vi "Main Development.vi"() -> ()   [LabVIEW 2021]
doc: "This template is for the Queued Message Handler design pattern.\n\nThe Event Handling Loop generates messages based on user interface actions.\n\nThe Message Handling Loop processes messages generated by the Event Handling Loop, or by other messages. The messages are string values, so new messages can be added easily to the Message Cases case structure in the Message Handling Loop. Each message cluster can also provide an optional value for Message Data, which is a variant that can be converted to whatever message-specific data is required."
uses:
  controls/UI Data.ctl
  support/Message Queue/Enqueue Message (Single).vi
  <vilib>/Utility/error.llb/Error Cluster From Error Code.vi
  <vilib>/ErrorRing/Error Ring.xnode
  support/Message Queue/Message Queue.lvlib
  support/User Event - Stop/User Event - Stop.lvlib
panel:
  out "Logging Clock":bool
  out "Sampling Clock":bool
  out "Logging Active":bool
  out "Log Delay":u32
  in  "Log Frequency (Hz)":dbl=2.0 min=0.0 step=1.0
  out "Sampling State":string(combo)="Paused"
  out "Pressure (bar)":dbl
  out "Pressure Chart":dbl(graph)
  out "Runtime Error out":errorcluster
  out "Measured Voltage":dbl format="%0.2f"
  out "Sample Delay mS":u32
  out "Logging State":string(combo)="Paused"
  out "Sampling Active":bool
  in  "Sample Rate (Hz)":dbl=10.0 min=0.0 step=1.0
  out "Program State":string
  in  "Start Logging":bool
  in  "Start Sampling":bool
  in  "Exit":bool
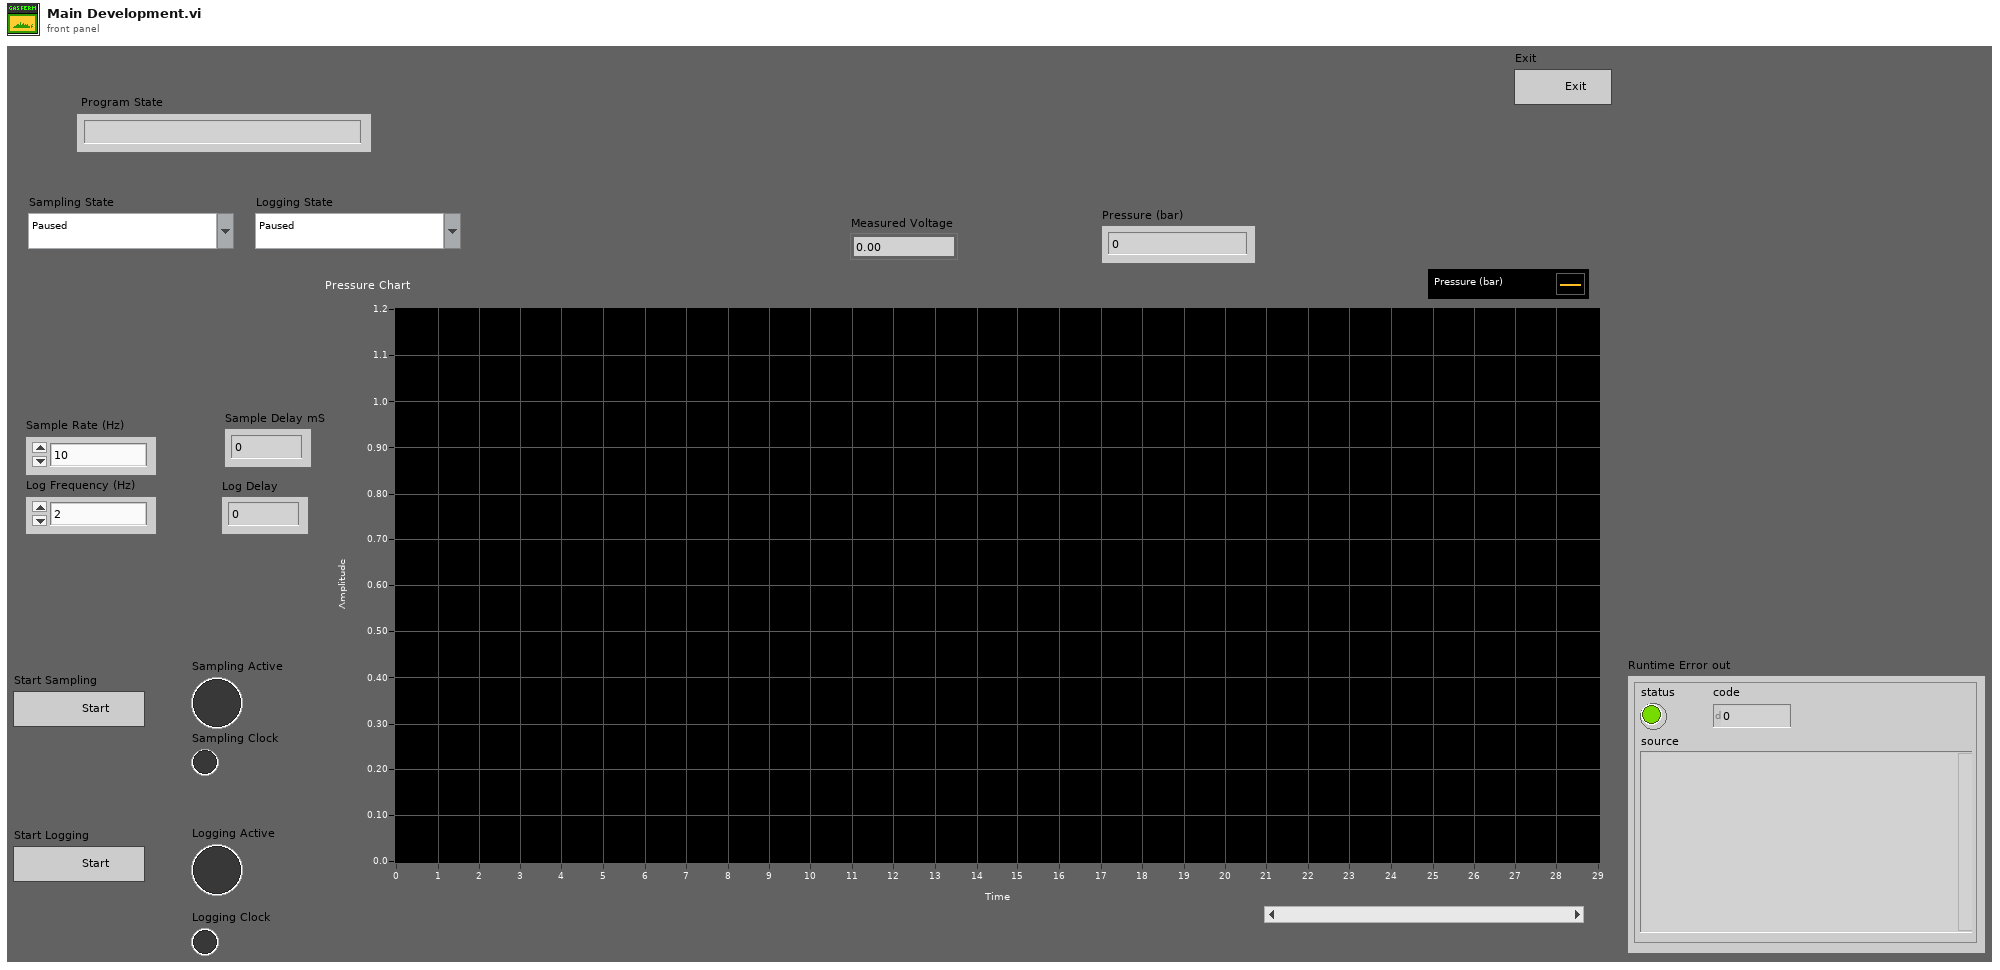
[diagram p1: front panel]
types:
  T1 = typedef "UI Data.ctl" = cluster{"Start Sampling":bool, "String <Replace Me>":string, "Numeric <Replace Me>":dbl, "Do Something Ref":refnum<vi>, "Do Something Else Ref":refnum<vi>, "Data Display Ref":refnum<vi>, "Exit Button Ref":refnum<vi>}
  T2 = typedef "Message Queue.lvlib/All Message Queues.ctl" = cluster{"UI":refnum<queue>}
  T3 = enum8{"Enabled", "Disabled", "Disabled and Grayed Out"}
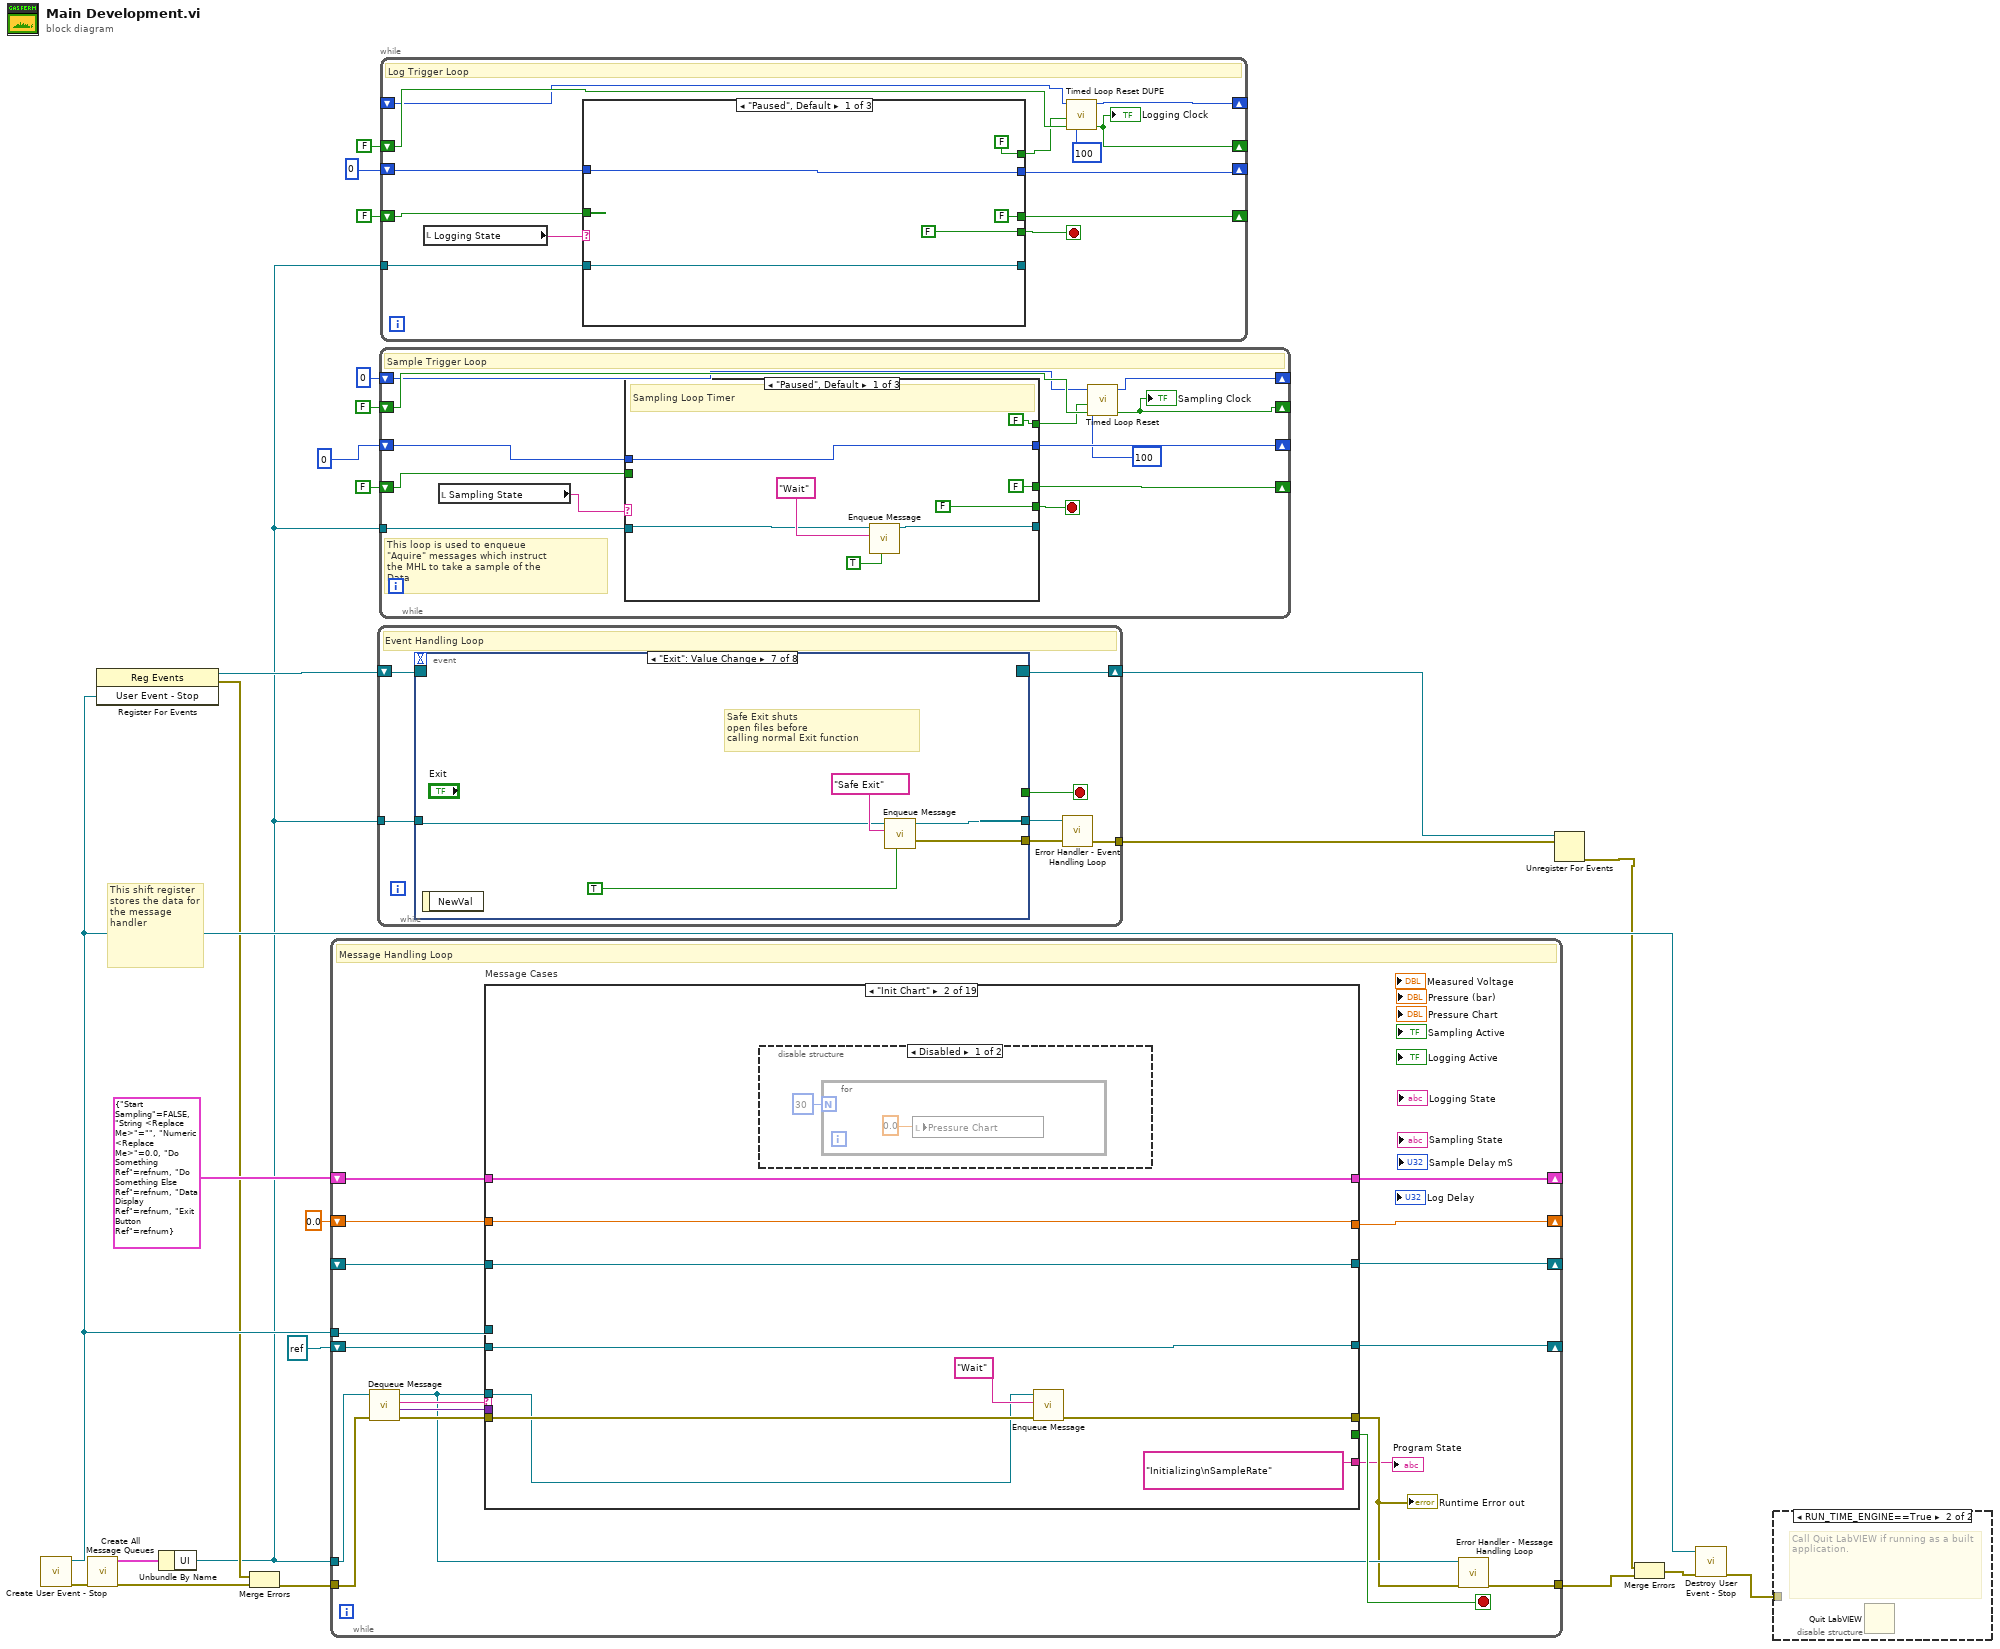
[diagram p0: block diagram]
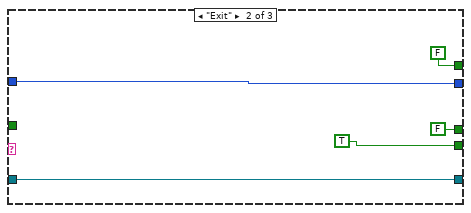
[diagram p2: hidden frame]
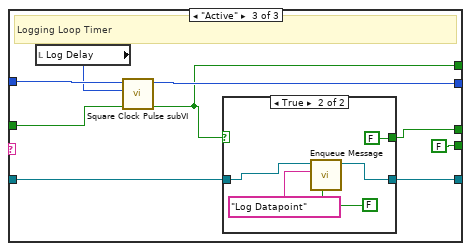
[diagram p3: hidden frame]
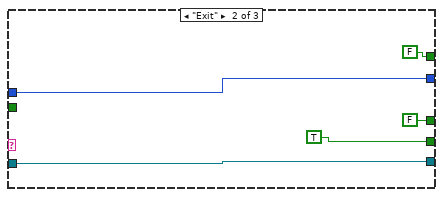
[diagram p5: hidden frame]
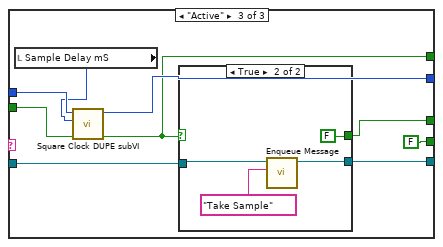
[diagram p6: hidden frame]
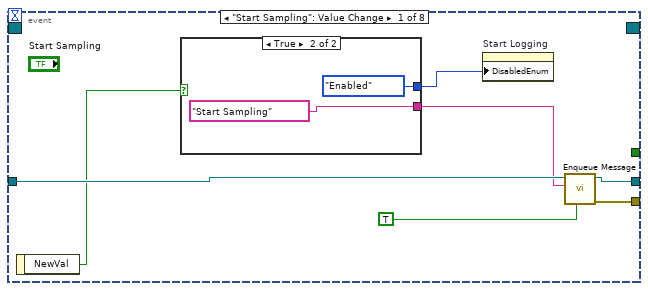
[diagram p9: hidden frame]
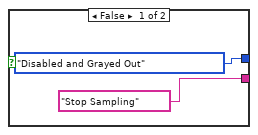
[diagram p10: hidden frame]
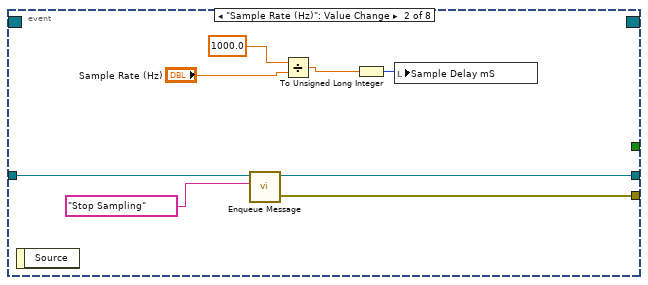
[diagram p11: hidden frame]
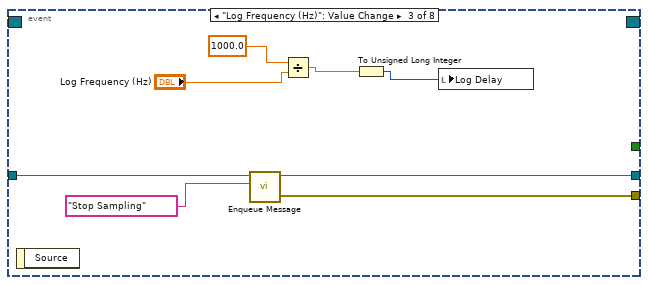
[diagram p12: hidden frame]
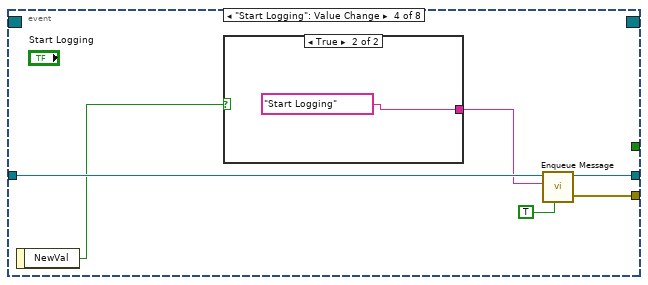
[diagram p13: hidden frame]
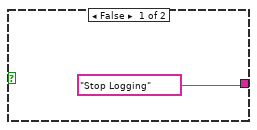
[diagram p14: hidden frame]
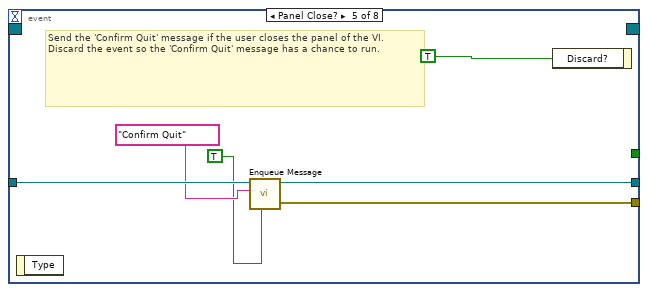
[diagram p15: hidden frame]
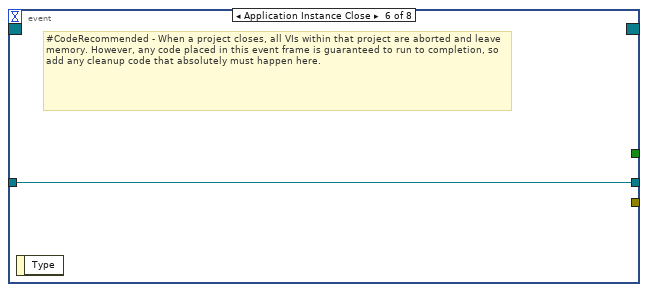
[diagram p16: hidden frame]
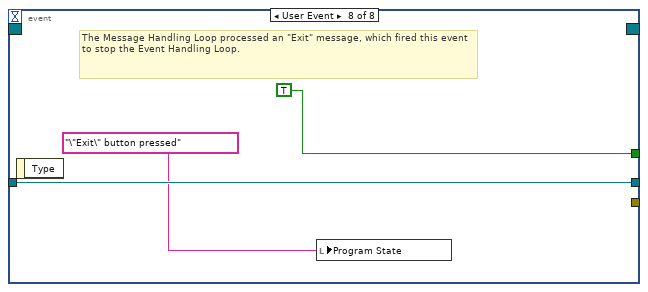
[diagram p17: hidden frame]
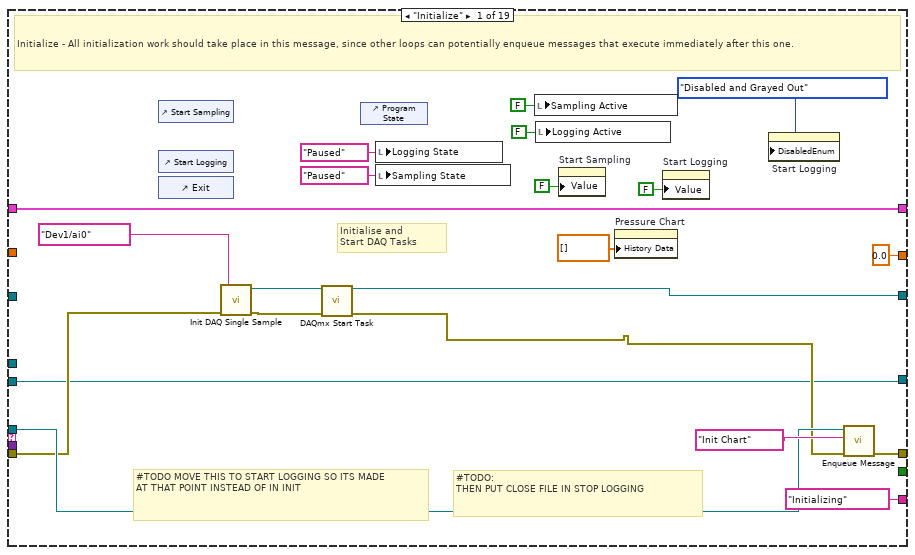
[diagram p18: hidden frame]
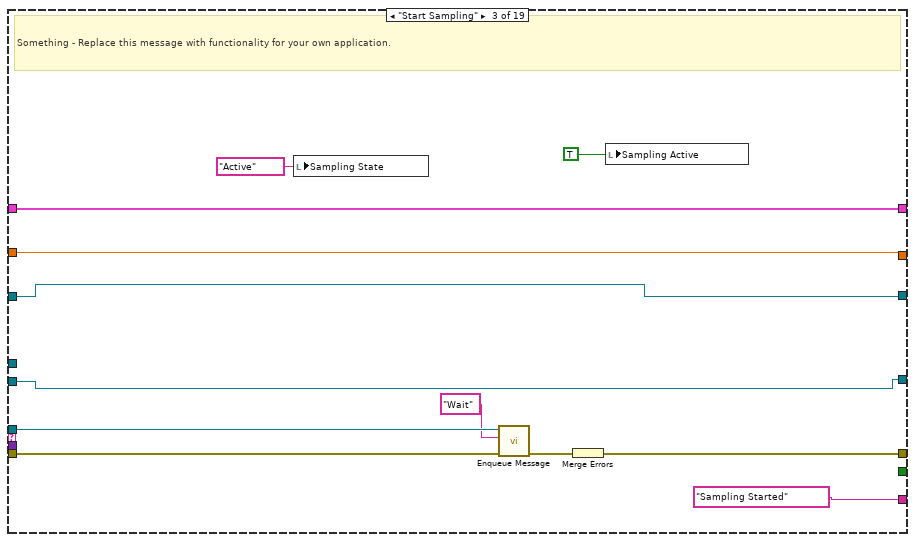
[diagram p20: hidden frame]
diagram:
  # "This shift register stores the data for the message handler"
  n1 = call "Create User Event - Stop.vi"() -> ("error out"=w22:errorcluster, "User Event - Stop"=w15:refnum<user-event>)  [unwired: 10 in]
  n2 = call "Create All Message Queues.vi"("error in (no error)"=w22) -> ("error out"=w24:errorcluster, "Message Queues out"=w23:T2)  [unwired: 9 in]
  n3 = register-events(w15) -> (reference out=w16:refnum<event-registration>, error out=w13:errorcluster)  [unwired: 2 in]
  n4 = Unbundle By Name(w23) -> ("UI"=w7:refnum<queue>)
  n5 = Merge Errors(w13, w24) -> (w14:errorcluster)
  n6 = while {
    tunnel: w7 -> [w35]
    shift-right: [w42] -> _
    shift-left: T1 {"Start Sampling"=FALSE, "String <Replace Me>"="", "Numeric <Replace Me>"=0.0, "Do Something Ref"=refnum, "Do Something Else Ref"=refnum, "Data Display Ref"=refnum, "Exit Button Ref"=refnum} ("Data Cluster") -> [w43]
    tunnel: w15 -> [w40]
    tunnel: w14 -> [w39]
    tunnel: [w33] -> w11
    shift-right: [w30] -> _
    shift-left: _ -> [w29]
    shift-right: [w28] -> _
    shift-left: refnum<file> refnum ("Byte Stream File out") -> [w27]
    shift-right: [w26] -> _
    shift-left: 0.0 ("Numeric Return") -> [w25]
    stop <- w41 stop-if-true
    # "Message Handling Loop"
    n7 = call "Dequeue Message.vi"("error in (no error)"=w39, "Message Queue"=w35) -> ("error out"=w38:errorcluster, "Message Data"=w36:variant, "Message"=w37:string, "dup Message Queue"=w34:refnum<queue>)  [unwired: 6 in]
    n8 = case "Message Cases" shown="\"Init Chart\"" w37 {
      selector: w37 -> [_ _ _ _ _ _ _ _ _ _ _ _ _ _ _ _ _ _ w292]
      tunnel: w34 -> [w62 w70 w83 w100 w110 w135 w152 w159 w182 w198 w205 w215 w226 _ _ w258 _ w287 _]
      tunnel: w38 -> [w56 w72 w85 w102 w111 w128 w145 w157 w178 w191 w207 w217 w228 w238 w251 w262 w269 w275 _]
      tunnel: [w64 w73 w86 w103 w116 w137 w154 w170 w179 w195 w208 w218 w229 w239 w245 w260 w267 w283 w293] -> w32
      tunnel: w43 -> [w60 w68 w87 w104 w117 w138 w155 w171 w183 w199 w209 w219 w230 w240 w250 w261 w268 w286 w294]
      tunnel: [w60 w68 w87 w104 w117 w138 w155 w171 w183 w199 w209 w219 w230 w240 w250 w261 w268 w286 w294] -> w42
      tunnel: [_ _ _ _ _ _ _ _ _ _ _ _ _ _ _ _ _ TRUE _] -> w41
      tunnel: w36 -> [_ _ _ _ _ _ _ _ _ _ _ _ _ w237 w249 _ _ w278 _]
      tunnel: w40 -> [_ _ _ _ _ _ _ _ _ _ _ _ _ _ _ _ _ w282 _]
      tunnel: ["Initializing" "Initializing\nSampleRate" "Sampling Started" "Logging Started" "Checking State" "Logging Stopped" "Safe Exit" "Sampling Stopped" "Taking Sample" "Logging Datapoint" "Paused" "Taking Sample" "Something Else" w234 "Error Detected" "Confirming Quit" "Waiting" "Exiting" "Invalid Message"] -> w31
      tunnel: [w57 w66 w79 w96 w112 w131 w148 w165 w177 w194 w202 w212 w221 w233 w243 w254 w265 w273 w290] -> w30
      tunnel: w29 -> [_ w66 w79 w96 w112 w131 w148 w165 w174 w194 w202 w212 w221 w233 w243 w254 w265 w273 w290]
      tunnel: [w52 w67 w78 w90 w113 refnum<file> refnum ("Byte Stream File out") refnum<file> refnum ("Byte Stream File out") w164 w175 w192 w201 w211 w222 w232 w242 w253 w264 w272 w289] -> w28
      tunnel: w27 -> [w52 w67 w78 _ w113 w129 w146 w164 w175 w193 w201 w211 w222 w232 w242 w253 w264 w272 w289]
      tunnel: [0.0 ("Numeric Return") w65 w77 w95 w114 w130 w147 0.0 ("Numeric Return") w172 w188 0.0 ("Numeric Return") w210 w220 w231 w241 w252 w263 0.0 ("Numeric Return") w288] -> w26
      tunnel: w25 -> [_ w65 w77 w95 w114 w130 w147 _ _ w189 _ w210 w220 w231 w241 w252 w263 _ w288]
      frame "Initialize" {
        # "#TODO:\nTHEN PUT CLOSE FILE IN STOP LOGGING"
        # "#TODO MOVE THIS TO START LOGGING SO ITS MADE\nAT THAT POINT INSTEAD OF IN INIT"
        # "Initialise and \nStart DAQ Tasks"
        # "Initialize - All initialization work should take place in this message, since other loops can potentially enqueue messages that execute immediately after this one."
        n9 = control-ref of="Start Sampling"() -> ()  [unwired: 1 out]
        n10 = control-ref of="Start Logging"() -> ()  [unwired: 1 out]
        n11 = control-ref of="Exit"() -> ()  [unwired: 1 out]
        n12 = call "Init DAQ Single Sample.vi"("error in"=w56, "physical channels"=tag "Dev1/ai0") -> ("error out"=w58:errorcluster, "Refnum out"=w59:refnum<k21>)  [unwired: 8 in]
        n13 = call <vilib>:"DAQmx Start Task.vi"("task/channels in"=w59, "error in"=w58) -> ("task out"=w57:refnum<k21>, "error out"=w53:errorcluster)  [unwired: 12 in]
        n14 = control-ref of="Program State"() -> ()  [unwired: 1 out]
        n15 = local write "Logging State"("Paused" ("Logging State")) -> ()
        n16 = local write "Sampling State"("Paused" ("Sampling State")) -> ()
        n17 = local write "Sampling Active"(FALSE ("Sampling Active")) -> ()
        n18 = local write "Logging Active"(FALSE ("Logging Active")) -> ()
        n19 = property on="Start Sampling" class="Bool (strict)"("Value"=FALSE ("Start Sampling")) -> ()  [unwired: 2 in, 2 out]
        n20 = property on="Pressure Chart" class="WFChart (strict)"("History Data"=dbl[] []) -> ()  [unwired: 2 in, 2 out]
        n21 = property on="Start Logging" class="Bool (strict)"("Value"=FALSE ("Start Logging")) -> ()  [unwired: 2 in, 2 out]
        n22 = property on="Start Logging" class="Bool (strict)"("DisabledEnum"=T3."Disabled and Grayed Out" ("Disabled")) -> ()  [unwired: 2 in, 2 out]
        n23 = call-poly "Enqueue Message.vi"("error in (no error)"=w53, "Message"="Init Chart", "Message Queue"=w62) -> ("error out"=w64:errorcluster)  [unwired: 7 in, 1 out]
      }
      frame "Init Chart" {
        n24 = disable-structure shown="Disabled" {
          frame Disabled {
            n25 = for {
              N: 30 -> [_]
              n26 = local write "Pressure Chart"(0.0 ("Pressure Chart")) -> ()
            }
          }
          frame Enabled {
          }
        }
        n27 = call-poly "Enqueue Message.vi"("error in (no error)"=w72, "Message"="Wait", "Message Queue"=w70) -> ("error out"=w73:errorcluster)  [unwired: 7 in, 1 out]
      }
      frame "Start Sampling" {
        # "Something - Replace this message with functionality for your own application."
        n28 = local write "Sampling State"("Active" ("Sampling State")) -> ()
        n29 = call-poly "Enqueue Message.vi"("error in (no error)"=w85, "Message"="Wait", "Message Queue"=w83) -> ("error out"=w84:errorcluster)  [unwired: 7 in, 1 out]
        n30 = Merge Errors(w84) -> (w86:errorcluster)
        n31 = local write "Sampling Active"(TRUE ("Sampling Active")) -> ()
      }
      frame "Start Logging" {
        w93 = "Time"  # Heading 1
        w94 = "Pressure"  # Heading 2
        w91 = "pressure-data"  # File Name
        w92 = path "Data"  # Relative Path or Folder
        # "Initialise and \nStart Log File"
        # "Something - Replace this message with functionality for your own application."
        n32 = local write "Logging Active"(TRUE ("Logging Active")) -> ()
        n33 = local write "Logging State"("Active" ("Sampling State")) -> ()
        n34 = call "Generate CSV File & Path with Headings.vi"("Heading 2"=w94, "Heading 1"=w93, "Relative Path or Folder"=w92, "File Name"=w91) -> ("error out"=w89:errorcluster, "Byte Stream File out"=w90:refnum<file>)  [unwired: 3 in, 3 out]
        n35 = call-poly "Enqueue Message.vi"("error in (no error)"=w102, "Message"="Wait", "Message Queue"=w100) -> ("error out"=w101:errorcluster)  [unwired: 7 in, 1 out]
        n36 = Merge Errors(w89, w101) -> (w103:errorcluster)
      }
      frame "Check Sampling" {
        # "Makes sure the system is in sampling mode if logging button is pressed"
        n37 = local read "Sampling State"() -> (w109:string)
        n38 = case shown="\"False\", Default" w109 {
          tunnel: w111 -> [w122 w123]
          tunnel: w110 -> [w120 w124]
          tunnel: [w119 w123] -> w108
          tunnel: [w118 w124] -> w106
          frame "False", Default {
            n39 = call-poly "Enqueue Message.vi"("error in (no error)"=w122, "Message"="Start Sampling", "Message Queue"=w120) -> ("error out"=w119:errorcluster, "dup Message Queue"=w118:refnum<queue>)  [unwired: 7 in]
          }
          frame "Active" {
          }
        }
        n40 = call-poly "Enqueue Message.vi"("error in (no error)"=w108, "Message"="Start Logging", "Message Queue"=w106) -> ("error out"=w107:errorcluster)  [unwired: 7 in, 1 out]
        n41 = Merge Errors(w107) -> (w116:errorcluster)
      }
      frame "Stop Logging" {
        # "#TODO Close Log File Here"
        # "Something - Replace this message with functionality for your own application."
        n42 = local write "Logging State"("Paused" ("Sampling State")) -> ()
        n43 = Close File(refnum=w129, error in=w128) -> (error out=w127:errorcluster)  [unwired: 1 out]
        n44 = local write "Logging Active"(FALSE ("Logging Active")) -> ()
        n45 = call-poly "Enqueue Message.vi"("error in (no error)"=w127, "Message"="Wait", "Message Queue"=w135) -> ("error out"=w136:errorcluster)  [unwired: 7 in, 1 out]
        n46 = Merge Errors(w136) -> (w137:errorcluster)
      }
      frame "Safe Exit" {
        # "Something - Replace this message with functionality for your own application."
        n47 = local write "Sampling State"("Paused" ("Sampling State")) -> ()
        n48 = local write "Logging State"("Paused" ("Sampling State")) -> ()
        n49 = local write "Sampling Active"(FALSE ("Sampling Active")) -> ()
        n50 = local write "Logging Active"(FALSE ("Logging Active")) -> ()
        n51 = Close File(refnum=w146, error in=w145) -> (error out=w144:errorcluster)  [unwired: 1 out]
        n52 = call-poly "Enqueue Message.vi"("Priority Message? (F)"=TRUE, "error in (no error)"=w144, "Message"="Exit", "Message Queue"=w152) -> ("error out"=w153:errorcluster)  [unwired: 6 in, 1 out]
        n53 = Merge Errors(w153) -> (w154:errorcluster)
      }
      frame "Stop Sampling" {
        # "Flush Queue because too many take sample que items?"
        n54 = local write "Sampling State"("Paused" ("Sampling State")) -> ()
        n55 = local write "Logging State"("Paused" ("Sampling State")) -> ()
        n56 = Flush Queue(queue=w159, error in (no error)=w157) -> (queue out=w158:refnum<queue>, error out=w156:errorcluster)  [unwired: 1 out]
        n57 = call-poly "Enqueue Message.vi"("error in (no error)"=w156, "Message"="Wait", "Message Queue"=w158) -> ("error out"=w169:errorcluster)  [unwired: 7 in, 1 out]
        n58 = local write "Sampling Active"(FALSE ("Sampling Active")) -> ()
        n59 = local write "Logging Active"(FALSE ("Logging Active")) -> ()
        n60 = Merge Errors(w169) -> (w170:errorcluster)
      }
      frame "Take Sample" {
        # "Example use of\nformula node"
        # "Next State \nto go to here"
        # "Something - Replace this message with functionality for your own application."
        n61 = call "Take Single Sample.vi"("error in (no error)"=w178, "Refnum in"=w174) -> ("error out"=w176:errorcluster, "Voltage Detected"=w173:dbl, "Refnum out"=w177:refnum<k21>)  [unwired: 7 in]
        n62 = local write "Measured Voltage"(w173) -> ()
        n63 = formula code="Pressure= Vin / 10;"("Vin"=w173) -> ("Pressure"=w172:dbl)
        n64 = local write "Pressure Chart"(w172) -> ()
        n65 = local write "Pressure (bar)"(w172) -> ()
        n66 = call-poly "Enqueue Message.vi"("error in (no error)"=w176, "Message"="Wait", "Message Queue"=w182) -> ("error out"=w179:errorcluster)  [unwired: 7 in, 1 out]
      }
      frame "Log Datapoint" {
        # "Next State \nto go to here"
        # "Something - Replace this message with functionality for your own application."
        n67 = call "Get Current DateTime.vi"("Leading Apostrophe"=FALSE, "Use Default String"=FALSE, "Date&Time format string (%c)"="%Y_%B_%d_%H:%M.%S") -> ("Date/Time String"=w184:string)  [unwired: 5 in, 3 out]
        n68 = call "Write Numeric to CSV File.vi"("error in (no error)"=w191, "Time String"=w184, "Numeric"=w189, "Byte Stream File in"=w193) -> ("error out"=w190:errorcluster, "Numeric Return"=w188:dbl, "Byte Stream File out"=w192:refnum<file>)  [unwired: 5 in]
        n69 = call-poly "Enqueue Message.vi"("error in (no error)"=w190, "Message"="Take Sample", "Message Queue"=w198) -> ("error out"=w195:errorcluster)  [unwired: 7 in, 1 out]
      }
      frame "Pause" {
        # "Something - Replace this message with functionality for your own application."
        n70 = call-poly "Enqueue Message.vi"("error in (no error)"=w207, "Message"="Indicator Off", "Message Queue"=w205) -> ("error out"=w206:errorcluster)  [unwired: 7 in, 1 out]
        n71 = Merge Errors(w206) -> (w208:errorcluster)
      }
      frame "Indicator Off" {
        # "Something - Replace this message with functionality for your own application."
        n72 = call-poly "Enqueue Message.vi"("error in (no error)"=w217, "Message"="Wait", "Message Queue"=w215) -> ("error out"=w216:errorcluster)  [unwired: 7 in, 1 out]
        n73 = Merge Errors(w216) -> (w218:errorcluster)
      }
      frame "Something Else" {
        # "Send string to \"Update Display\" message"
        # "#CodeNeeded - Perform whatever actions correspond to the \"Something Else\" message."
        # "Something Else - Replace this message with functionality for your own application."
        n74 = call-poly "Enqueue Message.vi"("error in (no error)"=w228, "Message Data"="\"Do Something Else\" button pressed" ("\"Do Something Else\" button pressed"), "Message"="Update Display", "Message Queue"=w226) -> ("error out"=w227:errorcluster)  [unwired: 6 in, 1 out]
        n75 = Merge Errors(w227) -> (w229:errorcluster)
      }
      frame "Update Display" {
        # "#CodeRecommended - If you wish to decouple the Message Handling Loop from your user interface, consider creating User Events (like the \"Stop\" event in this VI) to message the Event Handling Loop whenever the user interface needs updating."
        # "Update Display - Convert the message data to a string to display in the Data Display indicator."
        n76 = Variant To Data(error in=w238, type="", Variant=w237) -> (data=w234:string, error out=w235:errorcluster)
        n77 = Merge Errors(w235) -> (w239:errorcluster)
      }
      frame "Error" {
        # "#CodeRecommended - If you ever change the name of this \"Error\" message, you'll need to update the name in the Check Loop Error.vi as well."
        # "#CodeRecommended - Consider creating a system for logging errors in some way. These errors are for notification purposes only. Handling of specific errors should be performed in the message frames that generated the error."
        # "Error - Display an error dialog. This message is sent by the \"Error Handler\" VIs at the end of other loops in this application."
        n78 = Variant To Data(error in=w251, type=errorcluster {"status"=FALSE, "code"=0, "source"=""} ("error constant"), Variant=w249) -> (data=w247:errorcluster, error out=w246:errorcluster)
        n79 = call <vilib>:"Simple Error Handler.vi"("error in (no error)"=w247) -> ()  [unwired: 4 in, 5 out]
        n80 = Merge Errors(w246) -> (w245:errorcluster)
      }
      frame "Confirm Quit" {
        # "#CodeNeeded - If you want to provide an \"Are you sure\" dialog (or some other notification) before the application exits, place that code here. This message is typically sent from a Panel Close? event."
        # "Confirm Quit - Message that can confirm whether or not the user wants to exit the application."
        n81 = call-poly "Enqueue Message.vi"("Priority Message? (F)"=TRUE, "error in (no error)"=w262, "Message"="Exit", "Message Queue"=w258) -> ("error out"=w259:errorcluster)  [unwired: 6 in, 1 out]
        n82 = Merge Errors(w259) -> (w260:errorcluster)
      }
      frame "Wait" {
        # "Steady State - Waiting for command from event loop or trigger loop"
        n83 = Merge Errors(w269) -> (w267:errorcluster)
      }
      frame "Exit" {
        # "Stop the VI"
        # "Release the message queue reference"
        # "#CodeNeeded - Add any required cleanup code here. Note that if 'Exit' was called as a result of an error, an error dialog will be displayed. Add any custom error handling for an 'Exit' condition here as well."
        # "Exit - Exit the application."
        n84 = Variant To Data(type=errorcluster {"status"=FALSE, "code"=0, "source"=""} ("error constant"), Variant=w278) -> (data=w279:errorcluster)  [unwired: 1 in, 1 out]
        n85 = call <vilib>:"Simple Error Handler.vi"("error in (no error)"=w279) -> ()  [unwired: 4 in, 5 out]
        n86 = call <vilib>:"DAQmx Clear Task.vi"("task in"=w273, "error in"=w275) -> ("error out"=w274:errorcluster)  [unwired: 13 in]
        n87 = call "Fire User Event - Stop.vi"("User Event - Stop"=w282) -> ("error out"=w281:errorcluster)  [unwired: 10 in]
        n88 = Release Queue(queue=w287) -> (error out=w284:errorcluster)  [unwired: 2 in, 2 out]
        n89 = local write "Sampling State"("Exit" ("Sampling State")) -> ()
        n90 = local write "Logging State"("Exit" ("Sampling State")) -> ()
        n91 = Merge Errors(w281, w284, w274) -> (w283:errorcluster)
      }
      frame Default {
        # "'Default' case only runs if there is a message that isn't defined in any of the other cases.  Output a programming error."
        n92 = xnode "Error Ring"("parameter 0"=w292) -> ("error out"=w293:errorcluster)
      }
    }
    "Program State" <- w31
    "Runtime Error out" <- w32
    n93 = call "Error Handler - Message Handling Loop.vi"("error in (no error)"=w32, "Message Queue"=w34) -> ("dup error in"=w33:errorcluster)  [unwired: 8 in, 1 out]
  }
  n94 = while {
    tunnel: w7 -> [w308]
    shift-right: [w306] -> w20
    shift-left: w16 -> [w307]
    tunnel: [w302] -> w17
    stop <- w304 stop-if-true
    # "Event Handling Loop"
    n95 = event shown="[6] \"Exit\": Value Change" {
      selector: w307 -> [_ _ _ _ _ _ _ _]
      dyn-events: [_ _ _ _ _ _ _ _] -> w306
      timeout: _ -> [_ _ _ _ _ _ _ _]
      tunnel: [_ _ _ _ _ _ _ TRUE ("Discard?")] -> w304
      tunnel: w308 -> [w315 w327 w335 w341 w348 w350 w351 w358]
      tunnel: [w313 w325 w333 w339 w347 _ w355 _] -> w305
      tunnel: [w314 w326 w334 w340 w346 w350 w354 w358] -> w303
      event "Start Sampling": Value Change {
        n96 = event-data() -> ("NewVal"=w310:bool)  [unwired: 1 in]
        n97 = case shown="True" w310 {
          tunnel: ["Stop Sampling" ("Message") "Start Sampling" ("Message")] -> w312
          tunnel: [T3."Disabled and Grayed Out" ("Disabled") T3."Enabled" ("Disabled")] -> w309
          frame False {
          }
          frame True {
          }
        }
        n98 = property on="Start Logging" class="Bool (strict)"("DisabledEnum"=w309) -> ()  [unwired: 2 in, 2 out]
        n99 = call-poly "Enqueue Message.vi"("Priority Message? (F)"=TRUE, "Message"=w312, "Message Queue"=w315) -> ("error out"=w313:errorcluster, "dup Message Queue"=w314:refnum<queue>)  [unwired: 7 in]
      }
      event "Sample Rate (Hz)": Value Change {
        n100 = event-data() -> ()  [unwired: 1 in, 1 out]
        n101 = call-poly "Enqueue Message.vi"("Message"="Stop Sampling", "Message Queue"=w327) -> ("error out"=w325:errorcluster, "dup Message Queue"=w326:refnum<queue>)  [unwired: 8 in]
        n102 = Divide(x=1000.0, y="Sample Rate (Hz)") -> (x/y=w321:dbl)
        n103 = To Unsigned Long Integer(number=w321) -> (unsigned 32bit integer=w320:u32)
        n104 = local write "Sample Delay mS"(w320) -> ()
      }
      event "Log Frequency (Hz)": Value Change {
        n105 = event-data() -> ()  [unwired: 1 in, 1 out]
        n106 = call-poly "Enqueue Message.vi"("Message"="Stop Sampling", "Message Queue"=w335) -> ("error out"=w333:errorcluster, "dup Message Queue"=w334:refnum<queue>)  [unwired: 8 in]
        n107 = Divide(x=1000.0, y="Log Frequency (Hz)") -> (x/y=w330:dbl)
        n108 = To Unsigned Long Integer(number=w330) -> (unsigned 32bit integer=w328:u32)
        n109 = local write "Log Delay"(w328) -> ()
      }
      event "Start Logging": Value Change {
        n110 = event-data() -> ("NewVal"=w336:bool)  [unwired: 1 in]
        n111 = case shown="True" w336 {
          tunnel: ["Stop Logging" ("Message") "Start Logging" ("Message")] -> w338
          frame False {
          }
          frame True {
          }
        }
        n112 = call-poly "Enqueue Message.vi"("Priority Message? (F)"=TRUE, "Message"=w338, "Message Queue"=w341) -> ("error out"=w339:errorcluster, "dup Message Queue"=w340:refnum<queue>)  [unwired: 7 in]
      }
      event Panel Close? {
        # "Send the 'Confirm Quit' message if the user closes the panel of the VI. Discard the event so the 'Confirm Quit' message has a chance to run."
        n113 = event-data() -> ()  [unwired: 1 in, 1 out]
        n114 = call-poly "Enqueue Message.vi"("Priority Message? (F)"=TRUE, "Message"="Confirm Quit", "Message Queue"=w348) -> ("error out"=w347:errorcluster, "dup Message Queue"=w346:refnum<queue>)  [unwired: 7 in]
        n115 = event-data("Discard?"=TRUE) -> ()  [unwired: 1 in, 1 out]
      }
      event Application Instance Close {
        # "#CodeRecommended - When a project closes, all VIs within that project are aborted and leave memory. However, any code placed in this event frame is guaranteed to run to completion, so add any cleanup code that absolutely must happen here."
        n116 = event-data() -> ()  [unwired: 1 in, 1 out]
      }
      event "Exit": Value Change {
        # "Safe Exit shuts\nopen files before\ncalling normal Exit function"
        n117 = event-data() -> ()  [unwired: 1 in, 1 out]
        n118 = call-poly "Enqueue Message.vi"("Priority Message? (F)"=TRUE, "Message"="Safe Exit", "Message Queue"=w351) -> ("error out"=w355:errorcluster, "dup Message Queue"=w354:refnum<queue>)  [unwired: 7 in]
      }
      event User Event {
        # "The Message Handling Loop processed an \"Exit\" message, which fired this event to stop the Event Handling Loop."
        n119 = event-data() -> ()  [unwired: 1 in, 1 out]
        n120 = local write "Program State"("\"Exit\" button pressed" ("VI Stopped")) -> ()
      }
    }
    n121 = call "Error Handler - Event Handling Loop.vi"("error in (no error)"=w305, "Message Queue"=w303) -> ("dup error in"=w302:errorcluster)  [unwired: 8 in, 1 out]
  }
  n122 = while {
    tunnel: w7 -> [w371]
    shift-right: [w368] -> _
    shift-left: u32 0 ("Last Event mS") -> [w369]
    shift-right: [w360] -> _
    shift-left: FALSE -> [w366]
    shift-right: [w359] -> _
    shift-left: FALSE ("Bool Output") -> [w364]
    shift-right: [w362] -> _
    shift-left: u32 0 ("Last Event mS 2") -> [w361]
    stop <- w370 stop-if-true
    # "This loop is used to enqueue\n\"Aquire\" messages which instruct\nthe MHL to take a sample of the\nData"
    # "Sample Trigger Loop"
    n123 = local read "Sampling State"() -> (w367:string)
    n124 = case shown="\"Paused\", Default" w367 {
      tunnel: w371 -> [w376 w384 w392]
      tunnel: [w375 w384 w391] -> _
      tunnel: [FALSE TRUE FALSE] -> w370
      tunnel: w369 -> [w378 w382 w390]
      tunnel: [w378 w382 w389] -> w368
      tunnel: [FALSE FALSE w387] -> w360
      tunnel: w366 -> [_ _ w386]
      tunnel: [FALSE ("Clock Output") FALSE ("Clock Output") w385] -> w363
      frame "Paused", Default {
        # "Sampling Loop Timer"
        n125 = call-poly "Enqueue Message.vi"("Priority Message? (F)"=TRUE, "Message"="Wait", "Message Queue"=w376) -> ("dup Message Queue"=w375:refnum<queue>)  [unwired: 7 in, 1 out]
      }
      frame "Exit" {
      }
      frame "Active" {
        n126 = local read "Sample Delay mS"() -> (w388:u32)
        n127 = call "Square Clock DUPE subVI.vi"("Last Bool State"=w386, "SampleDelay(in)"=w388, "Last Event mS"=w390) -> ("Clock Output"=w385:bool, "Last Event mS"=w389:u32)  [unwired: 5 in, 2 out]
        n128 = case shown="True" w385 {
          selector: w385 -> [w394 _]
          tunnel: w392 -> [w395 w399]
          tunnel: [w395 w398] -> w391
          tunnel: [w394 FALSE] -> w387
          frame False {
          }
          frame True {
            n129 = call-poly "Enqueue Message.vi"("Message"="Take Sample", "Message Queue"=w399) -> ("dup Message Queue"=w398:refnum<queue>)  [unwired: 8 in, 1 out]
          }
        }
      }
    }
    n130 = call "Timed Loop Reset.vi"("Bool Current State"=w364, "Bool Set"=w363, "Trigger Time(mS)"=u32 100, "Last Event mS"=w361) -> ("Bool Output"=w359:bool, "Last Event mS 2"=w362:u32)  [unwired: 5 in, 1 out]
    "Sampling Clock" <- w359
  }
  n131 = while {
    shift-right: [w406] -> _
    shift-left: u32 0 ("Last Event mS") -> [w411]
    tunnel: w7 -> [w410]
    shift-right: [w407] -> _
    shift-left: FALSE -> [w408]
    shift-right: [w405] -> _
    shift-left: FALSE ("Bool Output") -> [w404]
    shift-right: [w402] -> _
    shift-left: _ -> [w401]
    stop <- w409 stop-if-true
    # "Log Trigger Loop"
    n132 = local read "Logging State"() -> (w412:string)
    n133 = case shown="\"Paused\", Default" w412 {
      tunnel: [w415 w420 w430] -> _
      tunnel: [FALSE TRUE FALSE] -> w409
      tunnel: [w416 w421 w428] -> w406
      tunnel: w411 -> [w416 w421 w429]
      tunnel: w410 -> [w415 w420 w427]
      tunnel: [FALSE FALSE w426] -> w407
      tunnel: w408 -> [_ _ w424]
      tunnel: [FALSE ("Clock Output") FALSE ("Clock Output") w423] -> w403
      frame "Paused", Default {
      }
      frame "Exit" {
      }
      frame "Active" {
        # "Logging Loop Timer"
        n134 = local read "Log Delay"() -> (w425:u32)
        n135 = call "Square Clock Pulse subVI.vi"("Last Bool State"=w424, "SampleDelay(in)"=w425, "Last Event mS"=w429) -> ("Clock Output"=w423:bool, "Last Event mS"=w428:u32)  [unwired: 5 in, 2 out]
        n136 = case shown="True" w423 {
          selector: w423 -> [w432 _]
          tunnel: [w433 w438] -> w430
          tunnel: w427 -> [w433 w435]
          tunnel: [w432 FALSE] -> w426
          frame False {
          }
          frame True {
            n137 = call-poly "Enqueue Message.vi"("Priority Message? (F)"=FALSE, "Message"="Log Datapoint", "Message Queue"=w435) -> ("dup Message Queue"=w438:refnum<queue>)  [unwired: 7 in, 1 out]
          }
        }
      }
    }
    n138 = call "Timed Loop Reset DUPE.vi"("Bool Current State"=w404, "Bool Set"=w403, "Trigger Time(mS)"=u32 100, "Last Event mS"=w401) -> ("Bool Output"=w405:bool, "Last Event mS 2"=w402:u32)  [unwired: 5 in, 1 out]
    "Logging Clock" <- w405
  }
  n139 = Unregister For Events(event registration refnum=w20, error in=w17) -> (error out=w9:errorcluster)
  n140 = Merge Errors(w9, w11) -> (w21:errorcluster)
  n141 = call "Destroy User Event - Stop.vi"("error in (no error)"=w21, "User Event - Stop"=w15) -> ("error out"=w18:errorcluster)  [unwired: 9 in]
  n142 = disable-structure shown="RUN_TIME_ENGINE==True" {
    disable-tunnel: w18 -> [_ _]
    frame condition #0 (active) {
    }
    frame condition #1 {
      # "Call Quit LabVIEW if running as a built application."
      n143 = Quit LabVIEW() -> ()  [unwired: 1 in]
    }
  }
